vi "Read Value.vi"(8 "error in (no error)":errorcluster, 11 "Block in":refnum<class "Block.lvclass">) -> (0 "error out":errorcluster, 2 "Value":u32, 3 "Block out":refnum<class "Block.lvclass">)   [LabVIEW 2016, in "Block.lvclass"]
uses:
  Block.lvclass
  Block.lvclass/Block.ctl
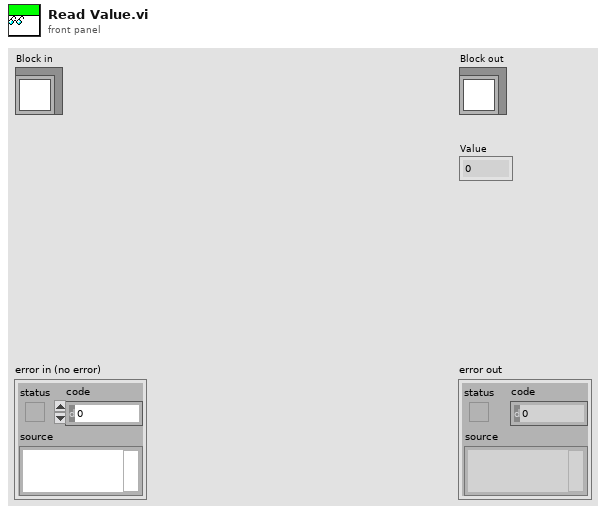
[diagram p1: front panel]
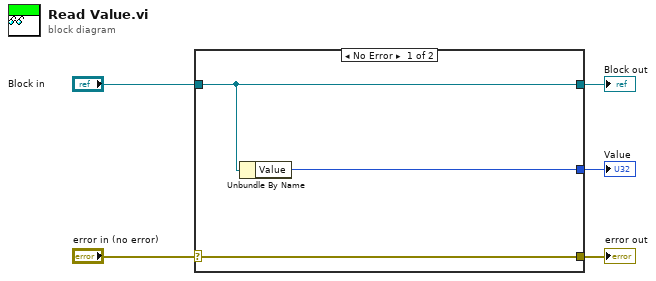
[diagram p0: block diagram]
diagram:
  n1 = case shown="No Error" "error in (no error)" {
    selector: "error in (no error)" -> [w8 w9]
    tunnel: [w8 w9] -> w4
    tunnel: [w7 w10] -> w2
    tunnel: "Block in" -> [w7 w10]
    tunnel: [w6 _] -> w1
    frame No Error {
      n2 = Unbundle By Name(w7) -> ("Value"=w6:u32)
    }
    frame Error {
    }
  }
  "error out" <- w4
  "Block out" <- w2
  "Value" <- w1
